vi "Actor Core.vi"(8 "error in":errorcluster, 11 "Main Display in":refnum<class "Main Display.lvclass">) -> (0 "error out":errorcluster, 3 "Actor out":refnum<class "Actor.lvclass">)   [LabVIEW 2016, in "Assert API Components.lvlib" / "Assert Display.lvlib" / "Main Display.lvlib" / "Main Display.lvclass"]
doc: "(<B>Filename</B>: Actor Framework.lvlib:Actor.lvclass:Actor Core.vi)\n\nReceives messages to the actor, reacts to them, and initiates any error handling that may shut the actor down.\n\nDescendant classes may override this VI to append parallel tasks for the actor to complete while it handles messages. Overrides use the Call Parent Method node."
uses:
  Main Display.lvclass
  C:/Program Files (x86)/National Instruments/LabVIEW 2016/vi.lib/ActorFramework/Actor/Actor.lvclass
  D:/Work/Projects/actor_assert_api/Core/Base UI Actor/Base UI Actor/Base UI Actor.lvclass
  D:/Work/Projects/actor_assert_api/Core/Base UI Component/Base UI Component/Base UI Component.lvclass
  <vilib>/ActorFramework/Actor/Actor.lvclass
  Display Colours.ctl
  Timing Engine/Timing Engine/Timing Engine.lvclass
  Main Display.lvclass/Main Display.ctl
  Base UI Component/Base UI Component/Base UI Component.lvclass/Base UI Component.ctl
  Base UI Actor/Base UI Actor/Base UI Actor.lvclass/Base UI Actor.ctl
  <vilib>/ActorFramework/Actor/Actor.lvclass/Actor.ctl
  <vilib>/ActorFramework/Message Enqueuer/Message Enqueuer.lvclass/Message Enqueuer.ctl
  Action Configuration.ctl
  Actions.ctl
  Main Display Messages/Do Action Msg/Do Action Msg.lvclass/Do Action Msg.ctl
  Main Display Messages/Set Display Colours Msg/Set Display Colours Msg.lvclass/Set Display Colours Msg.ctl
  Menu Click Data.ctl
  <vilib>/Utility/miscctls.llb/LVPoint32TypeDef.ctl
  Main Display Messages/Build Right Click Menu Msg/Build Right Click Menu Msg.lvclass/Build Right Click Menu Msg.ctl
  <vilib>/ActorFramework/Message Enqueuer/Init from Existing Queue.vi
  <vilib>/ActorFramework/Message Enqueuer/Enqueue.vi
  Main Display Messages/Do Action Msg/Do Action Msg.lvclass
  C:/Program Files (x86)/National Instruments/LabVIEW 2016/vi.lib/ActorFramework/Message/Message.lvclass
  Main Display Messages/Set Display Colours Msg/Set Display Colours Msg.lvclass
  Main Display Messages/Build Right Click Menu Msg/Build Right Click Menu Msg.lvclass
  <vilib>/ActorFramework/Message Priority Queue/Priority Enqueue.vi
  <vilib>/ActorFramework/Message Enqueuer/Message Enqueuer.lvclass
  Base UI Component/Base UI Component/Base UI Component.lvclass
  Right Click Menu Actions/RCM_Actions.lvclass
  Base UI Actor/Base UI Actor/Base UI Actor.lvclass
  Main Display.lvlib
panel:
  in  "Settings":bool
  in  "Main":bool
  out "Tab Control":enum32{"Display", "Settings"}(tab)
  in  "Assert Display Data":i32(listbox)
  in  "Display Colours":T1
  in  "Display Update Period":i32(slide)=1000 min=10 max=10000 scale=10.0..10000.0
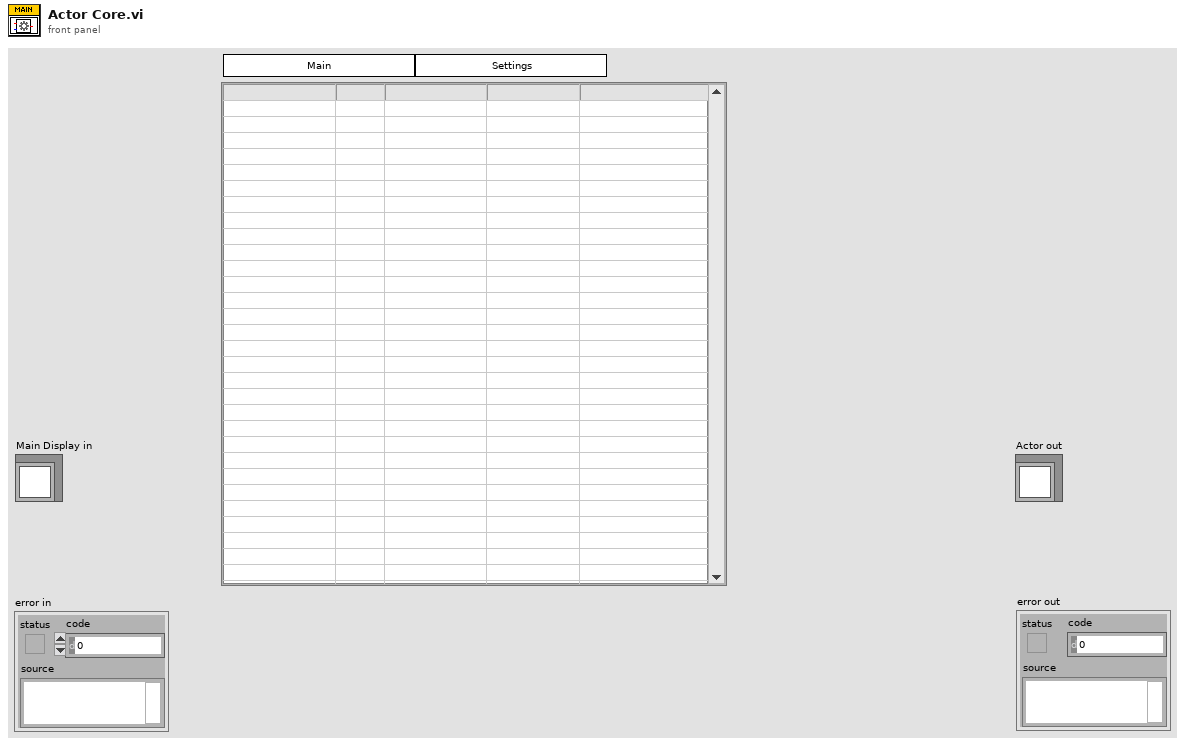
[diagram p1: front panel]
types:
  T1 = typedef "Assert API Components.lvlib/Assert Display.lvlib/Main Display.lvlib/Display Colours.ctl" = cluster{"Enable Colours":bool, "Passed Colour":u32, "Failed Colour":u32}
  T2 = typedef "Assert API Components.lvlib/Assert Display.lvlib/Main Display.lvlib/Menu Click Data.ctl" = cluster{"MenuRef":refnum<k9>, "Coords":T3, "Assert VI UID Array":i32[]}
  T3 = typedef "LVPoint32TypeDef.ctl" = cluster{"Horizontal":i32, "Vertical":i32}
  T4 = typedef "Assert API Components.lvlib/Assert Display.lvlib/Main Display.lvlib/Main Display.lvclass/Actions.ctl" = enum16{"Update Column Headers", "Update Timeout"}
  T5 = typedef "Assert API Components.lvlib/Assert Display.lvlib/Main Display.lvlib/Main Display.lvclass/Action Configuration.ctl" = cluster{"Action":T4, "Configuration":variant}
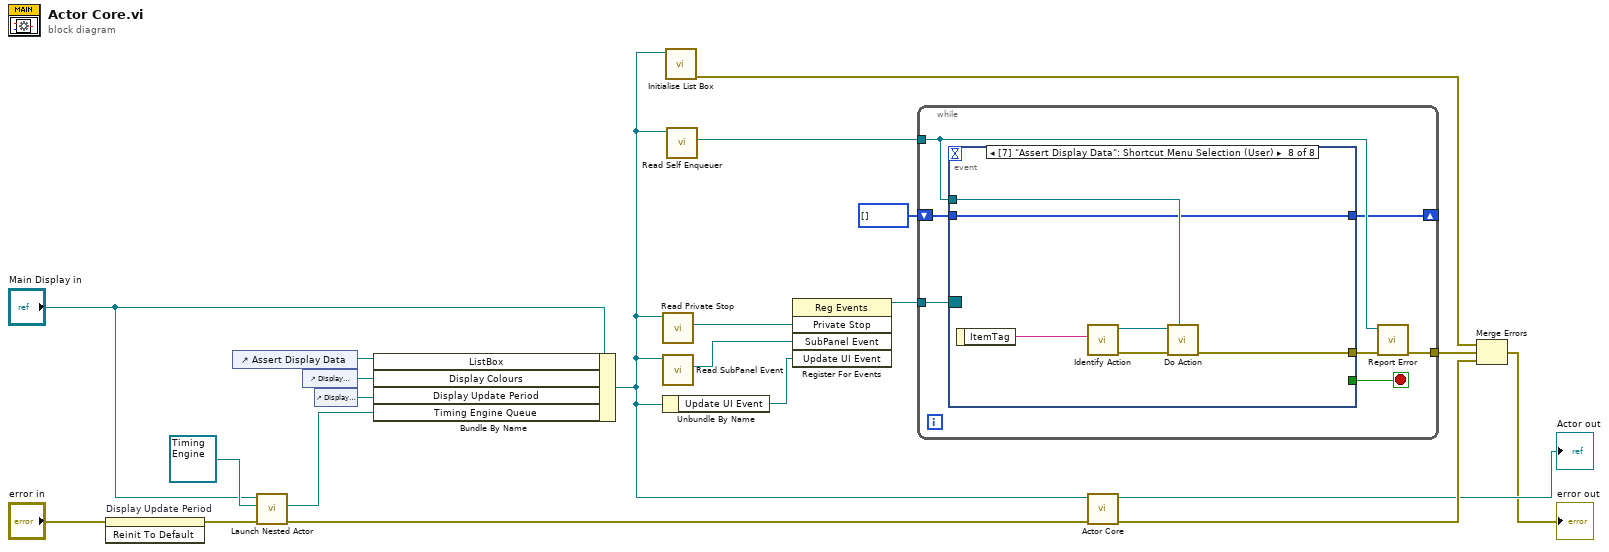
[diagram p0: block diagram]
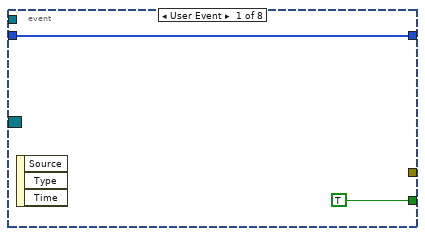
[diagram p2: hidden frame]
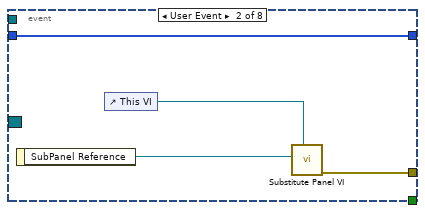
[diagram p3: hidden frame]
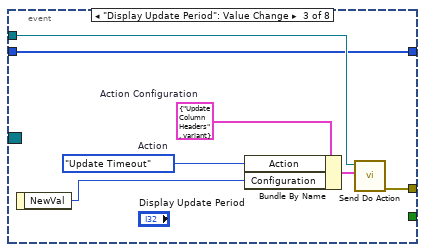
[diagram p4: hidden frame]
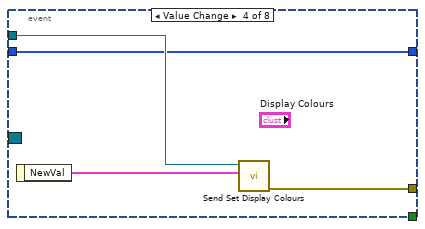
[diagram p5: hidden frame]
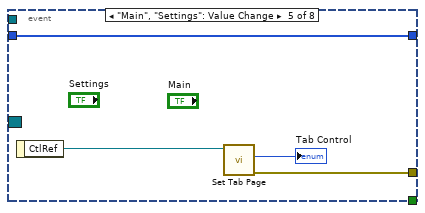
[diagram p6: hidden frame]
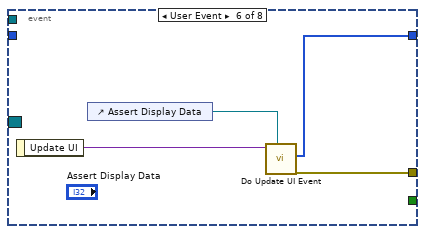
[diagram p7: hidden frame]
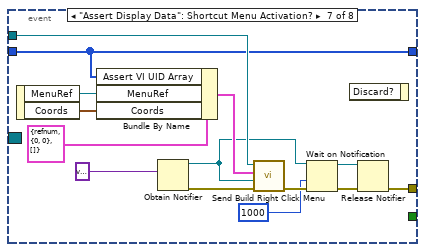
[diagram p8: hidden frame]
diagram:
  n1 = invoke on="Display Update Period" class="Slide (strict)" method="Reinit To Default"(error in="error in") -> (error out=w8:errorcluster)  [unwired: 2 in, 2 out]
  n2 = control-ref of="Assert Display Data"() -> (w4:refnum<vi>)
  n3 = call <vilib>:"Launch Nested Actor.vi"("error in (no error)"=w8, "Nested Actor"=refnum<class "Timing Engine.lvclass"> refnum ("Assert Display.lvlib:Timing Engine.lvlib:Timing Engine.lvclass"), "Caller Actor in"="Main Display in") -> ("error out"=w12:errorcluster, "Nested Actor's Enqueuer"=w13:refnum<class "Message Enqueuer.lvclass">)  [unwired: 6 in, 1 out]
  n4 = control-ref of="Display Colours"() -> (w3:refnum<vi>)
  n5 = control-ref of="Display Update Period"() -> (w2:refnum<vi>)
  n6 = Bundle By Name(cluster="Main Display in", "ListBox"=w4, "Display Colours"=w3, "Display Update Period"=w2, "Timing Engine Queue"=w13) -> (w5:refnum<class "Main Display.lvclass">)
  n7 = call "Read Private Stop.vi"("Base UI Actor in"=w5) -> ("Private Stop"=w19:refnum<user-event>)  [unwired: 10 in]
  n8 = call "Read SubPanel Event.vi"("Base UI Component in"=w5) -> ("SubPanel Event"=w18:refnum<user-event>)  [unwired: 10 in]
  n9 = Unbundle By Name(w5) -> ("Update UI Event"=w9:refnum<user-event>)
  n10 = call "Initialise List Box.vi"("Main Display in"=w5) -> ("error out"=w6:errorcluster)  [unwired: 10 in]
  n11 = call <vilib>:"Read Self Enqueuer.vi"("Actor"=w5) -> ("Self Enqueuer"=w7:refnum<class "Message Enqueuer.lvclass">)  [unwired: 10 in]
  n12 = register-events(w19, w18, w9) -> (reference out=w17:refnum<event-registration>)  [unwired: 2 in, 1 out]
  n13 = while {
    tunnel: w17 -> [w28]
    tunnel: [w25] -> w15
    tunnel: w7 -> [w24]
    shift-right: [w23] -> _
    shift-left: i32[] [] ("Assert VI UID Array") -> [w22]
    stop <- w26 stop-if-true
    n14 = event shown="[7] \"Assert Display Data\": Shortcut Menu Selection (User)" {
      selector: w28 -> [_ _ _ _ _ _ _ _]
      dyn-events: _ -> [_ _ _ _ _ _ _ _]
      timeout: _ -> [_ _ _ _ _ _ _ _]
      tunnel: [_ w34 w40 w43 w48 w53 w58 w70] -> w27
      tunnel: [TRUE _ _ _ _ _ _ _] -> w26
      tunnel: w24 -> [_ _ w41 w45 _ _ w66 w69]
      tunnel: [w29 w31 w35 w42 w46 w50 w54 w68] -> w23
      tunnel: w22 -> [w29 w31 w35 w42 w46 _ w54 w68]
      event User Event {
        n15 = event-data() -> ()  [unwired: 1 in, 3 out]
      }
      event User Event {
        n16 = event-data() -> ("SubPanel Reference"=w33:refnum<vi>)  [unwired: 1 in]
        n17 = control-ref of="This VI"() -> (w32:refnum<vi>)
        n18 = call "Substitute Panel VI.vi"("VI Reference"=w32, "SubPanel Reference"=w33) -> ("error out"=w34:errorcluster)  [unwired: 9 in]
      }
      event "Display Update Period": Value Change {
        w37 = Actions."Update Timeout"  # Action
        w39 = T5 {"Action"=enum."Update Column Headers", "Configuration"=variant}  # Action Configuration
        n19 = event-data() -> ("NewVal"=w36:i32)  [unwired: 1 in]
        n20 = Bundle By Name(cluster=w39, "Action"=w37, "Configuration"=w36) -> (w38:T5)
        n21 = call "Send Do Action.vi"("Action Configuration"=w38, "Message Enqueuer"=w41) -> ("error out"=w40:errorcluster)  [unwired: 8 in, 1 out]
      }
      event Value Change {
        n22 = event-data() -> ("NewVal"=w44:T1)  [unwired: 1 in]
        n23 = call "Send Set Display Colours.vi"("Display Colours"=w44, "Message Enqueuer"=w45) -> ("error out"=w43:errorcluster)  [unwired: 8 in, 1 out]
      }
      event "Main", "Settings": Value Change {
        n24 = event-data() -> ("CtlRef"=w49:refnum<vi>)  [unwired: 1 in]
        n25 = call "Set Tab Page.vi"("Control Reference in"=w49) -> ("error out"=w48:errorcluster, "Tab Control"=→"Tab Control":enum32{"Display", "Settings"})  [unwired: 9 in]
      }
      event User Event {
        n26 = event-data() -> ("Update UI"=w51:variant)  [unwired: 1 in]
        n27 = control-ref of="Assert Display Data"() -> (w52:refnum<vi>)
        n28 = call "Do Update UI Event.vi"("MulticolumnListbox in"=w52, "Update UI Data"=w51) -> ("error out"=w53:errorcluster, "Assert VI UID Array"=w50:i32[])  [unwired: 8 in]
      }
      event "Assert Display Data": Shortcut Menu Activation? {
        n29 = event-data() -> ("MenuRef"=w62:refnum<k9>, "Coords"=w61:T3)  [unwired: 1 in]
        n30 = Bundle By Name(cluster=T2 {"MenuRef"=refnum, "Coords"={"Horizontal"=0, "Vertical"=0}, "Assert VI UID Array"=[]} ("Menu Click Data"), "Assert VI UID Array"=w54, "MenuRef"=w62, "Coords"=w61) -> (w63:T2)
        n31 = Obtain Notifier(notification data type=variant) -> (notifier out=w56:refnum<notifier>, error out=w60:errorcluster)  [unwired: 3 in, 1 out]
        n32 = call "Send Build Right Click Menu.vi"("error in (no error)"=w60, "Return Notifier"=w56, "Menu Click Data"=w63, "Message Enqueuer"=w66) -> ("error out"=w67:errorcluster)  [unwired: 6 in, 1 out]
        n33 = Wait on Notification(notifier=w56, timeout in ms (-1)=1000, error in (no error)=w67) -> (notifier out=w57:refnum<notifier>, error out=w59:errorcluster)  [unwired: 1 in, 2 out]
        n34 = event-data() -> ()  [unwired: 2 in, 1 out]
        n35 = Release Notifier(notifier=w57, error in (no error)=w59) -> (error out=w58:errorcluster)  [unwired: 1 in, 2 out]
      }
      event "Assert Display Data": Shortcut Menu Selection (User) {
        n36 = event-data() -> ("ItemTag"=w73:string)  [unwired: 1 in]
        n37 = call "Identify Action.vi"("Item Tag"=w73) -> ("error out"=w71:errorcluster, "RCM_Actions out"=w72:refnum<class "RCM_Actions.lvclass">)  [unwired: 9 in]
        n38 = call-dynamic "Do Action.vi"("Self Enqueuer"=w69, "error in (no error)"=w71, "RCM_Actions in"=w72) -> ("error out"=w70:errorcluster)  [unwired: 8 in]
      }
    }
    n39 = call "Report Error.vi"("error in (no error)"=w27, "Self Enqueuer"=w24) -> ("error out"=w25:errorcluster)  [unwired: 9 in]
  }
  n40 = call-parent "Actor Core.vi"("error in"=w12, "Actor in"=w5) -> ("error out"=w21:errorcluster, "Actor out"=→"Actor out":refnum<class "Actor.lvclass">)  [unwired: 8 in]
  n41 = Merge Errors(w6, w15, w21) -> (→"error out":errorcluster)
